vi "geve-msg_macro_retry_serial_with_new_configuration.vi"(10 "Serial Port Configuration":T1={"timeout (ms)"=0, "VISA resource name"="", "baud rate"=0, "max expected byte count"=128}, 11 "Runtime Data in":T2) -> ()   [LabVIEW 2018]
doc: "send actions to retry serial com if it failed.\n- close serial\n- log message\n- update serial com\n- update config file\n- re-open serial port"
uses:
  geve-runtime_data_cluster.ctl
  geve-monitoring_data_cluster.ctl
  geve-serial_config_cluster.ctl
  geve-com_ref_cluster.ctl
  geve-message_cluster.ctl
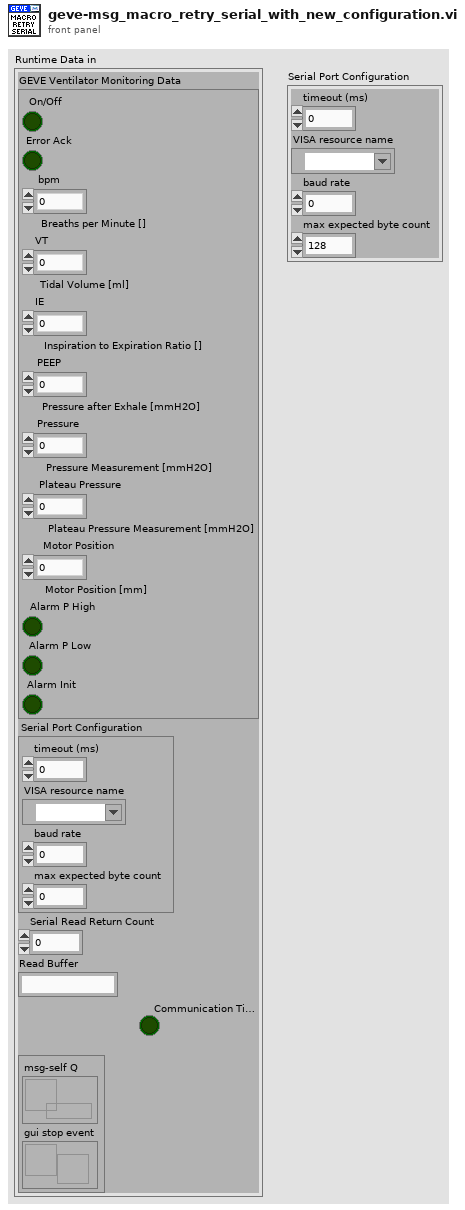
[diagram p1: front panel]
types:
  T1 = typedef "geve-serial_config_cluster.ctl" = cluster{"timeout (ms)":u32, "VISA resource name":refnum<visa-resource-name>, "baud rate":u32, "max expected byte count":u32}
  T2 = typedef "geve-runtime_data_cluster.ctl" = cluster{"GEVE Ventilator Monitoring Data":T3, "Serial Port Configuration":T1, "Serial Read Return Count":u32, "Read Buffer":string, "Communication Timeout?":bool, "com-refs":T4}
  T3 = typedef "geve-monitoring_data_cluster.ctl" = cluster{"On/Off":bool, "Error Ack":bool, "bpm":dbl, "VT":dbl, "IE":dbl, "PEEP":dbl, "Pressure":dbl, "Plateau Pressure":dbl, "Motor Position":dbl, "Alarm P High":bool, "Alarm P Low":bool, "Alarm Init":bool}
  T4 = typedef "geve-com_ref_cluster.ctl" = cluster{"msg-self Q":refnum<queue>, "gui stop event":refnum<user-event>}
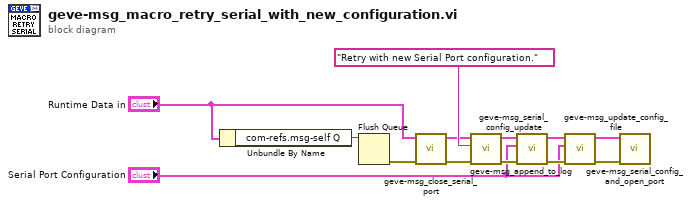
[diagram p0: block diagram]
diagram:
  n1 = Unbundle By Name("Runtime Data in") -> ("com-refs.msg-self Q"=w11:refnum<queue>)
  n2 = Flush Queue(queue=w11) -> (error out=w10:errorcluster)  [unwired: 1 in, 2 out]
  n3 = call "geve-msg_close_serial_port.vi"("error in (no error)"=w10, "Runtime Data"="Runtime Data in") -> ("error out"=w9:errorcluster, "Runtime Data out"=w7:T2)  [unwired: 8 in]
  n4 = call "geve-msg_append_to_log.vi"("error in (no error)"=w9, "Status Message"="Retry with new Serial Port configuration.", "Runtime Data"=w7) -> ("error out"=w12:errorcluster, "Runtime Dataout"=w6:T2)  [unwired: 7 in]
  n5 = call "geve-msg_serial_config_update.vi"("error in (no error)"=w12, "Serial Port Configuration"="Serial Port Configuration", "Runtime Data"=w6) -> ("error out"=w4:errorcluster, "Runtime Data out"=w5:T2)  [unwired: 7 in]
  n6 = call "geve-msg_update_config_file.vi"("error in (no error)"=w4, "Serial Port Configuration"="Serial Port Configuration", "Runtime Data"=w5) -> ("error out"=w3:errorcluster, "Runtime Data out"=w2:T2)  [unwired: 7 in]
  n7 = call "geve-msg_serial_config_and_open_port.vi"("error in (no error)"=w3, "Runtime Data"=w2) -> ()  [unwired: 8 in, 2 out]
